vi "Open.vi"(8 "error in (no error)":errorcluster, 10 "Update Rate (4Hz-100Hz)":u8=100, 11 "navX - SPI in":refnum<class "navX - SPI.lvclass">) -> (0 "error out":errorcluster, 3 "navX - SPI out":refnum<class "navX - SPI.lvclass">)   [LabVIEW 2015, in "navX Library v3.lvlib" / "navX - SPI.lvclass"]
uses:
  navX - SPI.lvclass
  navX - SPI.lvclass/navX - SPI.ctl
  navX - Base/navX - Base.lvclass
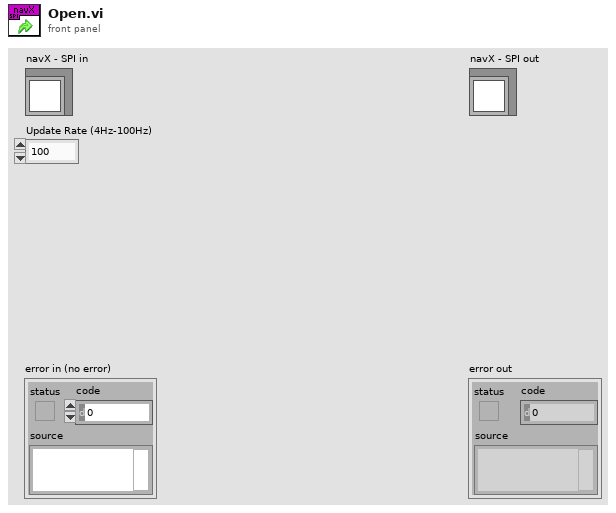
[diagram p1: front panel]
types:
  T1 = typedef "spi_bus.ctl" = enum16{"SPI On-Board, CS0", "SPI On-Board, CS1", "SPI On-Board, CS2", "SPI On-Board, CS3", "SPI MXP", "Invalid"}
  T2 = typedef "WPI_SPIDevRef.ctl" = cluster{"DevStatus":errorcluster, "Handle":i32, "SPI Bus":T1}
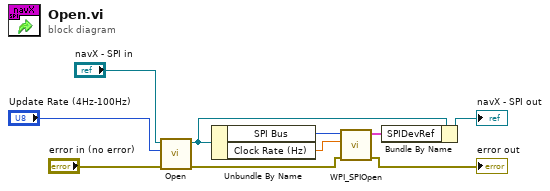
[diagram p0: block diagram]
diagram:
  n1 = call-parent "Open.vi"("error in (no error)"="error in (no error)", "Update Rate (4Hz-100Hz)"="Update Rate (4Hz-100Hz)", "navX - Base in"="navX - SPI in") -> ("error out"=w3:errorcluster, "navX - Base out"=w7:refnum<class "navX - SPI.lvclass">)  [unwired: 7 in]
  n2 = Unbundle By Name(w7) -> ("SPI Bus"=w5:T1, "Clock Rate (Hz)"=w4:dbl)
  n3 = call <vilib>:"WPI_SPIOpen.vi"("error in"=w3, "Clock Rate (Hz)"=w4, "SPI Bus"=w5) -> ("error out"=→"error out":errorcluster, "SPIDevRef"=w1:T2)  [unwired: 7 in]
  n4 = Bundle By Name(cluster=w7, "SPIDevRef"=w1) -> (→"navX - SPI out":refnum<class "navX - SPI.lvclass">)
